vi "Set Cells (1D Row DBL).vi"(6 "Column":i32, 7 "Values":dbl[](array[numeric]), 8 "error in (no error)":errorcluster, 9 "Row":i32, 10 "Sheet Reference":refnum<k24>) -> (0 "error out":errorcluster, 2 "Sheet Reference out":refnum<k24>)   [LabVIEW 2014]
uses:
  C:/PhaeronGit/LVNPOI/Resources/NPOI 2.1.1 dotnet2/NPOI.dll
  Resources/NPOI 2.1.1 dotnet2/NPOI.dll
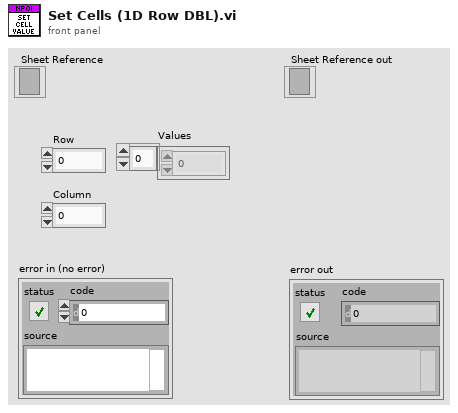
[diagram p1: front panel]
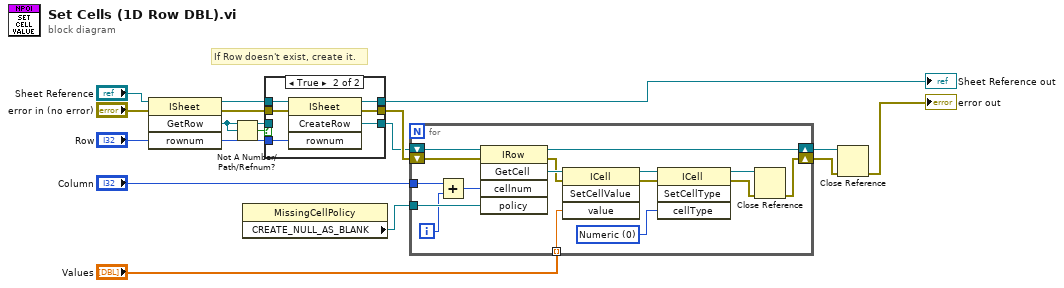
[diagram p0: block diagram]
diagram:
  # "If Row doesn't exist, create it."
  n1 = invoke class="ISheet" method="GetRow"(reference="Sheet Reference", error in="error in (no error)", "rownum"="Row") -> (reference out=w9:refnum<k24>, error out=w10:errorcluster, "GetRow"=w12:refnum<k24>)  [unwired: 1 in, 1 out]
  n2 = Not A Number/Path/Refnum?(number/path/refnum=w12) -> (NaN/Path/Refnum?=w11:bool)
  n3 = property class="MissingCellPolicy"() -> ("CREATE_NULL_AS_BLANK"=w2:refnum<k24>)  [unwired: 2 in, 2 out]
  n4 = case shown="True" w11 {
    tunnel: w9 -> [w19 w25]
    tunnel: w10 -> [w18 w24]
    tunnel: [w18 w23] -> w4
    tunnel: [w19 w22] -> w5
    tunnel: "Row" -> [_ w21]
    tunnel: [w17 w20] -> w3
    tunnel: w12 -> [w17 _]
    frame False {
    }
    frame True {
      n5 = invoke class="ISheet" method="CreateRow"(reference=w25, error in=w24, "rownum"=w21) -> (reference out=w22:refnum<k24>, error out=w23:errorcluster, "CreateRow"=w20:refnum<k24>)  [unwired: 1 in, 1 out]
    }
  }
  "Sheet Reference out" <- w5
  n6 = for {
    tunnel: "Column" -> [w40]
    tunnel: w2 -> [w34]
    shift-right: [w41] -> w16
    shift-left: w3 -> [w35]
    shift-right: [w37] -> w14
    shift-left: w4 -> [w36]
    tunnel: "Values" -> [w33] mode=indexing
    i -> [w31]
    w26 = 0 items=["Numeric"=0, "String"=1, "Formula"=2, "Blank"=3, "Boolean"=4, "Error"=5, "Unknown"=-1] ("cellType")
    n7 = Add(x=w40, y=w31) -> (x+y=w32:i32)
    n8 = invoke class="IRow" method="GetCell"(reference=w35, error in=w36, "cellnum"=w32, "policy"=w34) -> (reference out=w41:refnum<k24>, error out=w38:errorcluster, "GetCell"=w39:refnum<k24>)  [unwired: 1 in, 2 out]
    n9 = invoke class="ICell" method="SetCellValue"(reference=w39, error in=w38, "value"=w33) -> (reference out=w30:refnum<k24>, error out=w29:errorcluster)  [unwired: 1 in, 2 out]
    n10 = invoke class="ICell" method="SetCellType"(reference=w30, error in=w29, "cellType"=w26) -> (reference out=w28:refnum<k24>, error out=w27:errorcluster)  [unwired: 1 in, 2 out]
    n11 = Close Reference(reference=w28, error in (no error)=w27) -> (error out=w37:errorcluster)
  }
  n12 = Close Reference(reference=w16, error in (no error)=w14) -> (error out=→"error out":errorcluster)
